vi "_MobileTest_WriteReport.vi"(7 "Data":variant) -> ()   [LabVIEW 2019]
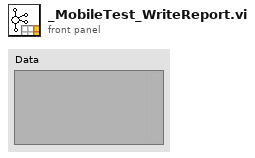
[diagram p1: front panel]
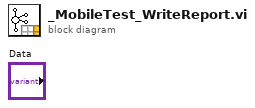
[diagram p0: block diagram]
diagram:
